vi "ChassisDriveDistance.vi"(8 "error in (no error)":errorcluster, 9 "RightDist":dbl, 10 "LeftDist":dbl) -> (0 "error out":errorcluster)   [LabVIEW 2014, in "ChassisLib.lvlib"]
uses:
  ChassisLib.lvlib
  <vilib>/addons/control/pid/pid.llb/PID (DBL).vi
  <vilib>/addons/control/pid/NI_PID_pid.lvlib
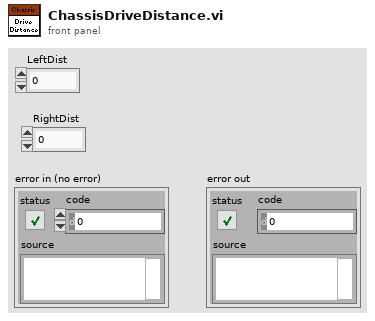
[diagram p1: front panel]
types:
  T1 = cluster{"proportional gain (Kc)":dbl, "integral time (Ti, min)":dbl, "derivative time (Td, min)":dbl}
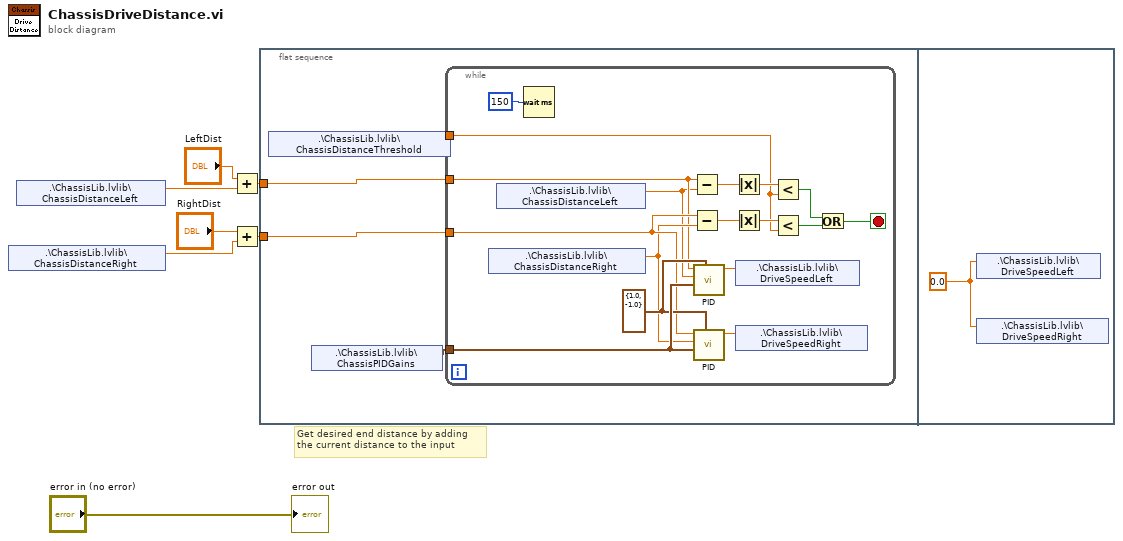
[diagram p0: block diagram]
diagram:
  # "Get desired end distance by adding \nthe current distance to the input"
  n1 = shared-variable ".\\ChassisLib.lvlib\\ChassisDistanceRight"() -> (w4:dbl)  [unwired: 1 in, 1 out]
  n2 = shared-variable ".\\ChassisLib.lvlib\\ChassisDistanceLeft"() -> (w6:dbl)  [unwired: 1 in, 1 out]
  n3 = Add(x="LeftDist", y=w6) -> (x+y=w3:dbl)
  n4 = Add(x="RightDist", y=w4) -> (x+y=w2:dbl)
  n5 = flat-sequence {
    tunnel: w3 -> [w10]
    tunnel: w2 -> [w9]
    frame #0 {
      n6 = shared-variable ".\\ChassisLib.lvlib\\ChassisDistanceThreshold"() -> (w8:dbl)  [unwired: 1 in, 1 out]
      n7 = shared-variable ".\\ChassisLib.lvlib\\ChassisPIDGains"() -> (w11:T1)  [unwired: 1 in, 1 out]
      n8 = while {
        tunnel: w11 -> [w27]
        tunnel: w10 -> [w17]
        tunnel: w9 -> [w23]
        tunnel: w8 -> [w12]
        stop <- w13 stop-if-true
        w26 = cluster{"output high":dbl, "output low":dbl} {"output high"=1.0, "output low"=-1.0} ("output range")
        n9 = shared-variable ".\\ChassisLib.lvlib\\ChassisDistanceRight"() -> (w22:dbl)  [unwired: 1 in, 1 out]
        n10 = shared-variable ".\\ChassisLib.lvlib\\ChassisDistanceLeft"() -> (w16:dbl)  [unwired: 1 in, 1 out]
        n11 = Wait (ms)(milliseconds to wait=u32 150) -> ()  [unwired: 1 out]
        n12 = Subtract(x=w17, y=w16) -> (x-y=w18:dbl)
        n13 = Subtract(x=w23, y=w22) -> (x-y=w21:dbl)
        n14 = call-poly <vilib>:"PID.vi"("output range"=w26, "PID gains"=w27, "process variable"=w16, "setpoint"=w17) -> ("output"=w25:dbl)  [unwired: 6 in, 1 out]
        n15 = call-poly <vilib>:"PID.vi"("output range"=w26, "PID gains"=w27, "process variable"=w22, "setpoint"=w23) -> ("output"=w24:dbl)  [unwired: 6 in, 1 out]
        n16 = Absolute Value(x=w18) -> (abs(x)=w19:dbl)
        n17 = Absolute Value(x=w21) -> (abs(x)=w20:dbl)
        n18 = shared-variable ".\\ChassisLib.lvlib\\DriveSpeedLeft"(w25) -> ()  [unwired: 1 in, 1 out]
        n19 = shared-variable ".\\ChassisLib.lvlib\\DriveSpeedRight"(w24) -> ()  [unwired: 1 in, 1 out]
        n20 = Less?(x=w19, y=w12) -> (x < y?=w14:bool)
        n21 = Less?(x=w20, y=w12) -> (x < y?=w15:bool)
        n22 = Or(x=w14, y=w15) -> (x .or. y?=w13:bool)
      }
    }
    frame #1 {
      w29 = 0.0
      n23 = shared-variable ".\\ChassisLib.lvlib\\DriveSpeedLeft"(w29) -> ()  [unwired: 1 in, 1 out]
      n24 = shared-variable ".\\ChassisLib.lvlib\\DriveSpeedRight"(w29) -> ()  [unwired: 1 in, 1 out]
    }
  }
  "error out" <- "error in (no error)"
